vi "ToTable.vi"(8 "error in (no error)":errorcluster, 9 "Table Index":i32, 10 "variant":variant, 11 "node in":refnum<class "TDMS datalogger editor node.lvclass">) -> (0 "error out":errorcluster, 1 "row header":string[](array[string]), 2 "table":string[][](array[string]), 3 "node in out":refnum<class "TDMS datalogger editor node.lvclass">)   [LabVIEW 2015, in "TDMS datalogger editor node.lvclass"]
doc: "Copyright 2017 National Instruments Corporation\n\nLicensed under the Apache License, Version 2.0 (the \"License\"); you may not use this file except in compliance with the License. You may obtain a copy of the License at http://www.apache.org/licenses/LICENSE-2.0\nUnless required by applicable law or agreed to in writing, software distributed under the License is distributed on an \"AS IS\" BASIS, WITHOUT WARRANTIES OR CONDITIONS OF ANY KIND, either express or implied. See the License for the specific language governing permissions and limitations under the License."
uses:
  <vilib>/NI/DCAF/Modules/TDMSModule/editor/TDMS datalogger editor node.lvclass
  <vilib>/NI/Tag Bus/tag/tag descriptor.lvclass
  <vilib>/NI/Module Execution Interface/Engine Configuration/engine configuration.lvclass
  <vilib>/NI/Tag Bus Module Framework/channel/TBM channel.lvclass
  <vilib>/NI/Configuration Framework/serializable configuration/NISE_CEF_serializable configuration.lvclass
  <vilib>/NI/DCAF/Modules/TDMSModule/module/configuration/TDMS datalogger configuration.lvclass
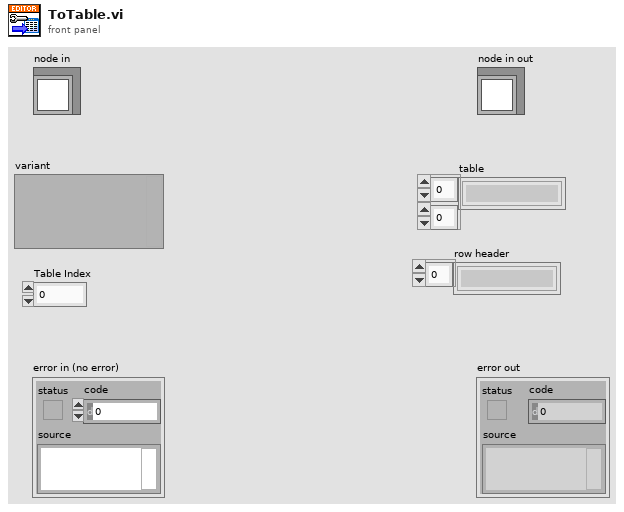
[diagram p1: front panel]
types:
  T1 = cluster{"channel":refnum<class "TBM channel.lvclass">}[]
  T2 = typedef "TBM channel.lvclass/channel classification.ctl" = enum16{"input data", "output data", "processing parameter", "processing result"}
  T3 = typedef "tag bus.lvlib/tag descriptor.lvclass/Data Type.ctl" = enum16{"Double", "Single", "I64", "I32", "I16", "I8", "U64", "U32", "U16", "U8", "Boolean", "String", "Array of Double", "Array of Single", "Array of I64", "Array of I32", "Array of I16", "Array of I8", "Array of U64", "Array of U32", "Array of U16", "Array of U8", "Array of Boolean", "Array of String"}
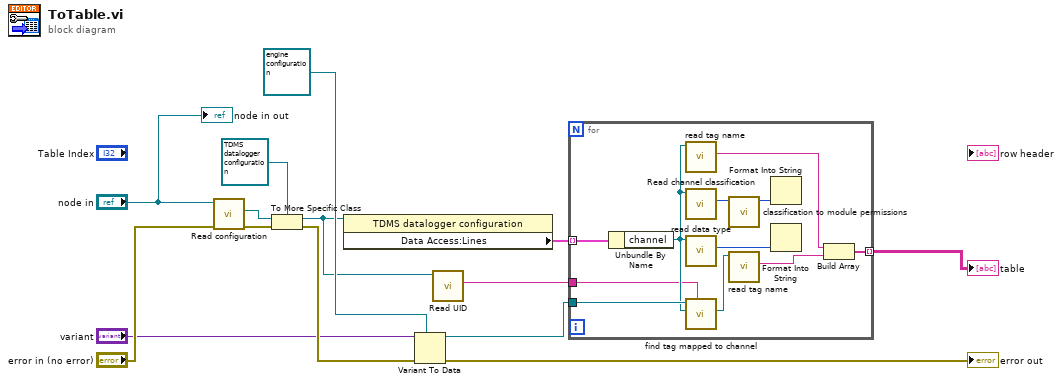
[diagram p0: block diagram]
diagram:
  n1 = call-dynamic "Read configuration.vi"("error in"="error in (no error)", "TDMS datalogger editor node in"="node in") -> ("error out"=w14:errorcluster, "configuration"=w10:refnum<class "NISE_CEF_serializable configuration.lvclass">)  [unwired: 7 in, 1 out]
  n2 = To More Specific Class(target class=refnum<class "TDMS datalogger configuration.lvclass"> refnum ("TDMS datalogger configuration"), reference=w10, error in=w14) -> (specific class reference=w9:refnum<class "TDMS datalogger configuration.lvclass">, error out=w7:errorcluster)
  n3 = property on="Property Node" class="TDMS datalogger configuration"(reference=w9) -> ("Data Access:Lines"=w13:T1)  [unwired: 1 in, 2 out]
  n4 = Variant To Data(error in=w7, type=refnum<class "engine configuration.lvclass"> refnum ("engine configuration"), Variant="variant") -> (data=w12:refnum<class "engine configuration.lvclass">, error out=→"error out":errorcluster)
  n5 = call <vilib>:"Read UID.vi"("configuration in"=w9) -> ("instance id"=w8:string)  [unwired: 8 in, 2 out]
  n6 = for {
    tunnel: w13 -> [w25] mode=indexing
    tunnel: w12 -> [w23]
    tunnel: [w16] -> w4 mode=indexing
    tunnel: w8 -> [w15]
    n7 = Unbundle By Name(w25) -> ("channel"=w18:refnum<class "TBM channel.lvclass">)
    n8 = call <vilib>:"read tag name.vi"("system tag in"=w18) -> ("name"=w24:string)  [unwired: 8 in, 2 out]
    n9 = call <vilib>:"Read channel classification.vi"("channel in"=w18) -> ("channel classification"=w21:T2)  [unwired: 8 in, 2 out]
    n10 = call <vilib>:"read data type.vi"("system tag in"=w18) -> ("data type"=w17:T3)  [unwired: 8 in, 2 out]
    n11 = call <vilib>:"find tag mapped to channel.vi"("owner"=w15, "channel"=w18, "engine configuration in"=w23) -> ("tag"=w22:refnum<class "tag descriptor.lvclass">)  [unwired: 6 in, 2 out]
    n12 = call <vilib>:"classification to module permissions.vi"("channel classification"=w21) -> ("view direction"=w20:enum32{"Read from HW", "Write to HW"})  [unwired: 10 in]
    n13 = call <vilib>:"read tag name.vi"("system tag in"=w22) -> ("name"=w19:string)  [unwired: 8 in, 2 out]
    n14 = Format Into String(w20) -> ()  [unwired: 3 in, 2 out]
    n15 = Format Into String(w17) -> ()  [unwired: 3 in, 2 out]
    n16 = Build Array(w24, w19) -> (w16:string[])
  }
  "table" <- w4
  "node in out" <- "node in"
